vi "Permute_Array.vi"(9 "permute_rule":i32[](array[numeric]), 10 "Input_Dims":i32[](array[numeric]), 11 "1D Array In":sgl[](array[numeric])) -> (2 "Permuted_Dims":i32[](array[numeric]), 3 "1D Array out":sgl[](array[numeric]))   [LabVIEW 2020]
panel:
  # "rr"
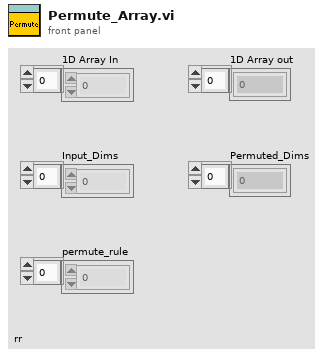
[diagram p1: front panel]
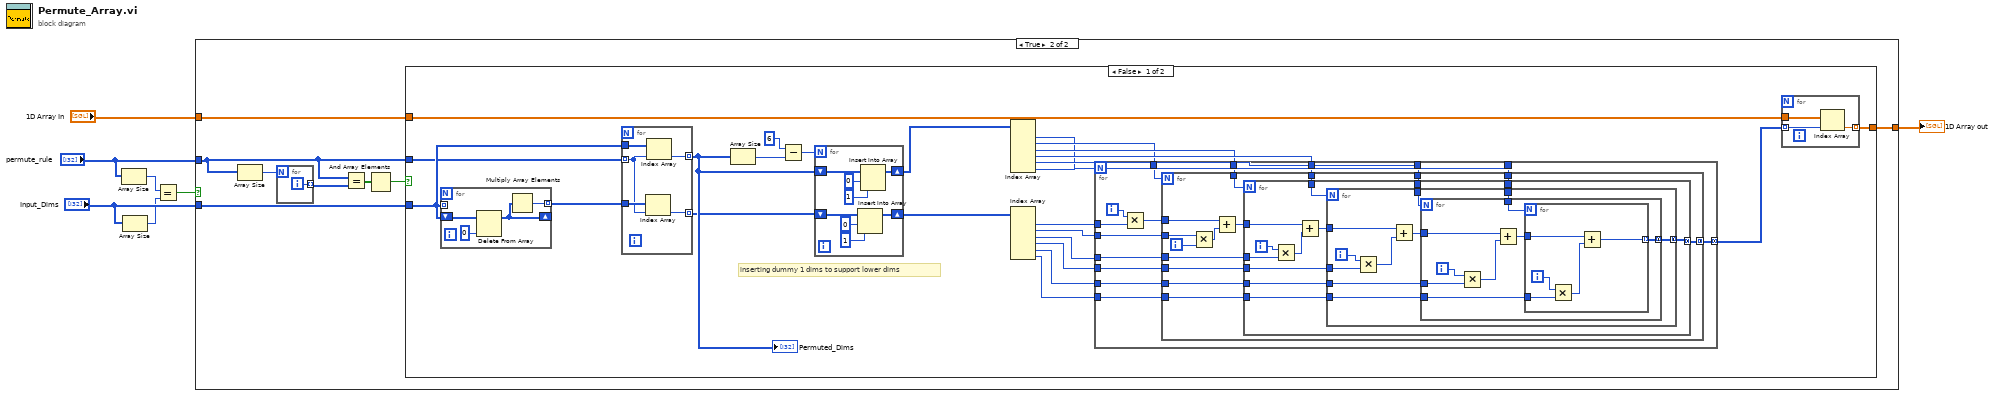
[diagram p0: block diagram]
diagram:
  n1 = Array Size(array="permute_rule") -> (size(s)=w3:i32)
  n2 = Array Size(array="Input_Dims") -> (size(s)=w2:i32)
  n3 = Equal?(x=w3, y=w2) -> (x = y?=w1:bool)
  n4 = case shown="True" w1 {
    tunnel: [_ w15] -> w7
    tunnel: "1D Array In" -> [_ w14]
    tunnel: "permute_rule" -> [_ w12]
    tunnel: "Input_Dims" -> [_ w13]
    frame False {
    }
    frame True {
      n5 = Array Size(array=w12) -> (size(s)=w10:i32)
      n6 = for {
        N: w10 -> [_]
        tunnel: [w125] -> w11 mode=indexing
        i -> [w125]
      }
      n7 = Equal?(x=w12, y=w11) -> (x = y?=w9:bool[])
      n8 = And Array Elements(Boolean array=w9) -> (logical AND=w8:bool)
      n9 = case shown="False" w8 {
        tunnel: [w20 w124] -> w15
        tunnel: w14 -> [w19 w124]
        tunnel: w13 -> [w17 _]
        tunnel: w12 -> [w16 _]
        frame False {
          # "inserting dummy 1 dims to support lower dims"
          n10 = for {
            tunnel: w17 -> [_] mode=indexing
            tunnel: [w122] -> w37 mode=indexing
            shift-right: [w121] -> _
            shift-left: w17 -> [w123]
            n11 = Delete From Array(array=w123, index=0) -> (array with subset deleted=w121:i32[])  [unwired: 1 in, 1 out]
            n12 = Multiply Array Elements(1:w121) -> (0:w122:i32)
          }
          n13 = for {
            tunnel: w16 -> [w108] mode=indexing
            tunnel: w17 -> [w111]
            tunnel: [w110] -> w40 mode=indexing
            tunnel: w37 -> [w109]
            tunnel: [w107] -> w36 mode=indexing
            n14 = Index Array(array=w109, index=w108) -> (element=w107:i32)
            n15 = Index Array(array=w111, index=w108) -> (element=w110:i32)
          }
          "Permuted_Dims" <- w40
          n16 = Array Size(array=w40) -> (size(s)=w33:i32)
          n17 = Subtract(x=6 ("y"), y=w33) -> (x-y=w34:i32)
          n18 = for {
            N: w34 -> [_]
            shift-right: [w119] -> w39
            shift-left: w40 -> [w118]
            shift-right: [w113] -> w38
            shift-left: w36 -> [w112]
            n19 = Insert Into Array(array=w112, index=0, new element=1 ("new element/subarray")) -> (w113:i32[])
            n20 = Insert Into Array(array=w118, index=0, new element=1 ("new element/subarray")) -> (w119:i32[])
          }
          n21 = Index Array(array=w39) -> (element #1=w21:i32, element #2=w22:i32, element #3=w29:i32, element #4=w30:i32, element #5=w31:i32, element #6=w32:i32)  [unwired: 6 in]
          n22 = Index Array(array=w38) -> (element #1=w23:i32, element #2=w25:i32, element #3=w24:i32, element #4=w26:i32, element #5=w27:i32, element #6=w28:i32)  [unwired: 6 in]
          n23 = for {
            N: w21 -> [_]
            tunnel: w22 -> [w57]
            tunnel: w29 -> [w56]
            tunnel: w23 -> [w54]
            tunnel: w25 -> [w53]
            tunnel: w24 -> [w52]
            tunnel: [w50] -> w18 mode=concatenating
            tunnel: w26 -> [w49]
            tunnel: w27 -> [w48]
            tunnel: w28 -> [w47]
            tunnel: w30 -> [w46]
            tunnel: w31 -> [w45]
            tunnel: w32 -> [w44]
            i -> [w55]
            n24 = Multiply(x=w55, y=w54) -> (x*y=w51:i32)
            n25 = for {
              N: w57 -> [_]
              tunnel: w56 -> [w71]
              tunnel: w53 -> [w69]
              tunnel: w52 -> [w68]
              tunnel: w51 -> [w65]
              tunnel: [w64] -> w50 mode=concatenating
              tunnel: w49 -> [w63]
              tunnel: w48 -> [w62]
              tunnel: w47 -> [w61]
              tunnel: w46 -> [w60]
              tunnel: w45 -> [w59]
              tunnel: w44 -> [w58]
              i -> [w70]
              n26 = Multiply(x=w69, y=w70) -> (x*y=w67:i32)
              n27 = Add(x=w65, y=w67) -> (x+y=w66:i32)
              n28 = for {
                N: w71 -> [_]
                tunnel: w68 -> [w82]
                tunnel: w66 -> [w80]
                tunnel: [w75] -> w64 mode=concatenating
                tunnel: w63 -> [w78]
                tunnel: w62 -> [w77]
                tunnel: w61 -> [w76]
                tunnel: w60 -> [w74]
                tunnel: w59 -> [w73]
                tunnel: w58 -> [w72]
                i -> [w83]
                n29 = Multiply(x=w83, y=w82) -> (x*y=w81:i32)
                n30 = Add(x=w80, y=w81) -> (x+y=w79:i32)
                n31 = for {
                  N: w74 -> [_]
                  tunnel: w79 -> [w90]
                  tunnel: w78 -> [w91]
                  tunnel: w77 -> [w88]
                  tunnel: w76 -> [w87]
                  tunnel: [w86] -> w75 mode=concatenating
                  tunnel: w73 -> [w85]
                  tunnel: w72 -> [w84]
                  i -> [w92]
                  n32 = Multiply(x=w92, y=w91) -> (x*y=w93:i32)
                  n33 = Add(x=w90, y=w93) -> (x+y=w89:i32)
                  n34 = for {
                    N: w85 -> [_]
                    tunnel: w89 -> [w100]
                    tunnel: w88 -> [w99]
                    tunnel: w87 -> [w96]
                    tunnel: [w95] -> w86 mode=concatenating
                    tunnel: w84 -> [w94]
                    i -> [w98]
                    n35 = Multiply(x=w98, y=w99) -> (x*y=w101:i32)
                    n36 = Add(x=w100, y=w101) -> (x+y=w97:i32)
                    n37 = for {
                      N: w94 -> [_]
                      tunnel: w97 -> [w105]
                      tunnel: w96 -> [w103]
                      tunnel: [w102] -> w95 mode=indexing
                      i -> [w104]
                      n38 = Multiply(x=w104, y=w103) -> (x*y=w106:i32)
                      n39 = Add(x=w105, y=w106) -> (x+y=w102:i32)
                    }
                  }
                }
              }
            }
          }
          n40 = for {
            tunnel: w19 -> [w43]
            tunnel: [w42] -> w20 mode=indexing
            tunnel: w18 -> [w41] mode=indexing
            n41 = Index Array(array=w43, index=w41) -> (element=w42:sgl)
          }
        }
        frame True {
        }
      }
    }
  }
  "1D Array out" <- w7
